vi "SpecAn Select and Initiate Measurements.vi"(0 "Instrument Handle In":refnum<k21>, 1 "Selector String":string, 2 "Result Name":string, 5 "Measurements":T1(array[ring]), 7 "Auto Level Configuration":T2={"Enabled"=FALSE, "Measurement Interval (s)"=0.01} {"Measurement Interval (s)" min=1e-06 max=100.0 format="%.2p"}, 9 "Auto Level Bandwidth (Hz)":dbl=200000.0 format="%.6p", 11 "error in (no error)":errorcluster, 12 "Enable All Traces (F)":bool) -> (4 "Instrument Handle Out":refnum<k21>, 6 "Selector String Out":string, 15 "error out":errorcluster)   [LabVIEW 2019, in "RFmxSpecAn.lvlib"]
doc: "Performs actions to initiate acquisition and measurement. \n\nEnables the specified measurement(s) before optionally automatically adjusting the reference level before beginning measurements. Finally, initiates the acquisition and measurement(s)."
uses:
  RFmxSpecAn.lvlib
  Common/SA Auto Level Configuration.ctl
  <vilib>/RFmx/SpecAn/mx/RFmxSpecAn.llb/RFmxSpecAn Select Measurement (Multiple).vi
  Common/Common.lvlib
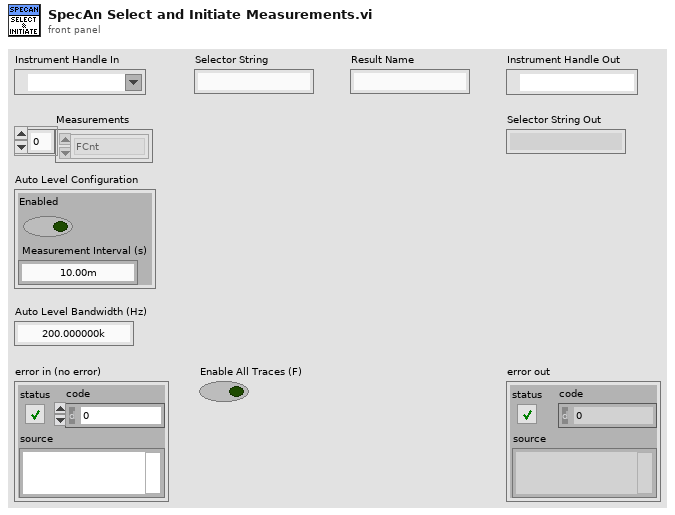
[diagram p1: front panel]
types:
  T1 = enum16{"ACP", "CCDF", "CHP", "FCnt", "Harmonics", "OBW", "SEM", "Spectrum", "Spur", "TXP", "AMPM", "DPD", "IQ", "IM", "NF", "PhaseNoise", "PAVT"}[]
  T2 = typedef "Common.lvlib/SA Auto Level Configuration.ctl" = cluster{"Enabled":bool, "Measurement Interval (s)":dbl}
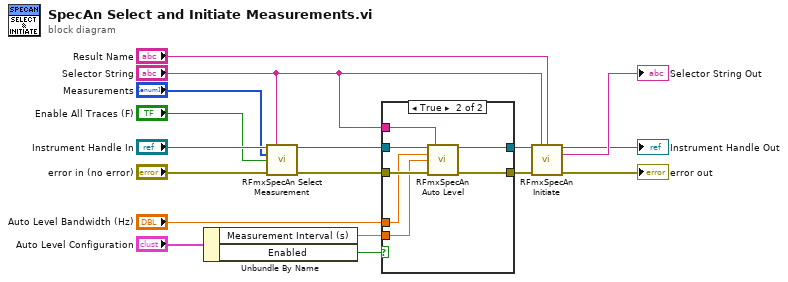
[diagram p0: block diagram]
diagram:
  n1 = Unbundle By Name("Auto Level Configuration") -> ("Measurement Interval (s)"=w4:dbl, "Enabled"=w5:bool)
  n2 = call-poly <vilib>:"RFmxSpecAn Select Measurement.vi"("Instrument Handle In"="Instrument Handle In", "Selector String"="Selector String", "Measurements"="Measurements", "Enable All Traces"="Enable All Traces (F)", "error in (no error)"="error in (no error)") -> ("Instrument Handle Out"=w8:refnum<k21>, "error out"=w14:errorcluster)  [unwired: 9 in]
  n3 = case shown="True" w5 {
    tunnel: w14 -> [w18 w26]
    tunnel: [w18 w25] -> w9
    tunnel: w8 -> [w19 w24]
    tunnel: [w19 w23] -> w7
    tunnel: w4 -> [_ w22]
    tunnel: "Selector String" -> [_ w21]
    tunnel: "Auto Level Bandwidth (Hz)" -> [_ w20]
    frame False {
    }
    frame True {
      n4 = call <vilib>:"RFmxSpecAn Auto Level.vi"("Instrument Handle In"=w24, "Selector String"=w21, "Bandwidth (Hz)"=w20, "Measurement Interval (s)"=w22, "error in (no error)"=w26) -> ("Instrument Handle Out"=w23:refnum<k21>, "error out"=w25:errorcluster)  [unwired: 8 in, 1 out]
    }
  }
  n5 = call <vilib>:"RFmxSpecAn Initiate.vi"("Instrument Handle In"=w7, "Selector String"="Selector String", "Result Name"="Result Name", "error in (no error)"=w9) -> ("Instrument Handle Out"=→"Instrument Handle Out":refnum<k21>, "Selector String Out"=→"Selector String Out":string, "error out"=→"error out":errorcluster)  [unwired: 9 in]
